vi "get_safe_path.vi"(7 "filename":string, 8 "error in":errorcluster, 9 "num_points":i32, 10 "end_label":string, 11 "start_label":string) -> (0 "error out":errorcluster, 1 "coordinate_list":sgl[](array[numeric]), 2 "num_points out":i32)   [LabVIEW 2011, in "gVision.lvlib"]
uses:
  gVision.lvlib
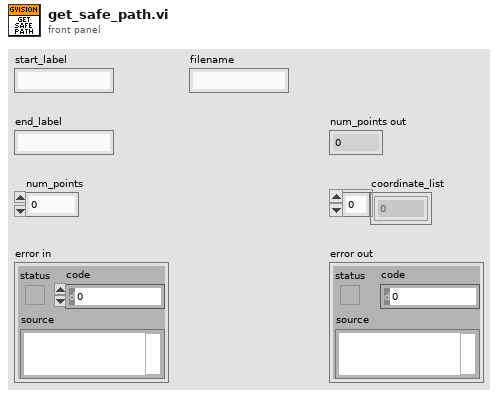
[diagram p1: front panel]
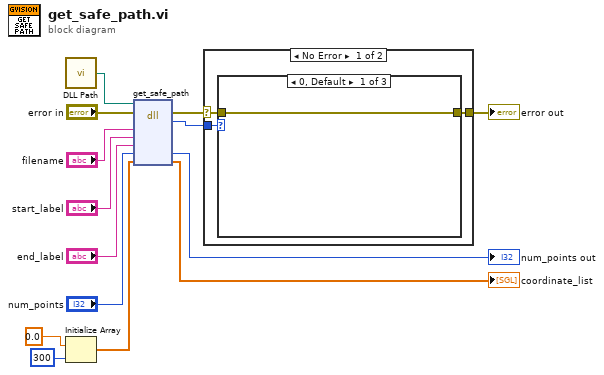
[diagram p0: block diagram]
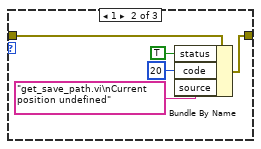
[diagram p2: hidden frame]
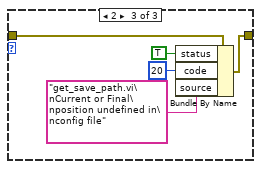
[diagram p3: hidden frame]
diagram:
  n1 = call "DLL Path.vi"() -> ("DLL Path"=w4:path)  [unwired: 5 in]
  n2 = Initialize Array(sgl 0.0 ("element"), 300 ("dimension size")) -> (w12:sgl[])
  n3 = dll-call lib="?" fn="get_safe_path"(path in=w4, error in="error in", "filename"="filename", "start_label"="start_label", "end_label"="end_label", "num_points"="num_points", "coordinate_list"=w12) -> (error out=w3:errorcluster, "error code"=w2:i32, "num_points"=→"num_points out":i32, "coordinate_list"=→"coordinate_list":sgl[])  [unwired: 4 in, 1 out]
  n4 = case shown="No Error" w3 {
    selector: w3 -> [w16 w29]
    tunnel: w2 -> [w17 _]
    tunnel: [w15 w29] -> w1
    frame No Error {
      n5 = case shown="0, Default" w17 {
        tunnel: w16 -> [w18 w23 w25]
        tunnel: [w18 w22 w24] -> w15
        frame 0, Default {
        }
        frame 1 {
          n6 = Bundle By Name(cluster=w23, "status"=TRUE, "code"=20, "source"="get_save_path.vi\nCurrent position undefined") -> (w22:errorcluster)
        }
        frame 2 {
          n7 = Bundle By Name(cluster=w25, "status"=TRUE, "code"=20, "source"="get_save_path.vi\nCurrent or Final\nposition undefined in\nconfig file") -> (w24:errorcluster)
        }
      }
    }
    frame Error {
    }
  }
  "error out" <- w1
